vi "Release.vi"(8 "error in (no error)":errorcluster, 11 "[User] Cfg File in":refnum<class "[User] Cfg File.lvclass">) -> (0 "error out":errorcluster, 3 "[User] Cfg File out":refnum<class "[User] Cfg File.lvclass">)   [LabVIEW 2020, in "[User] Cfg File.lvclass"]
uses:
  [User] Cfg File.lvclass
  [User] Cfg File.lvclass/[User] Cfg File.ctl
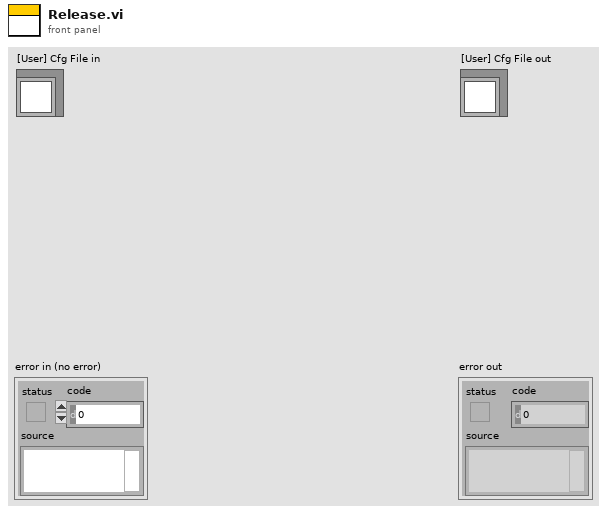
[diagram p1: front panel]
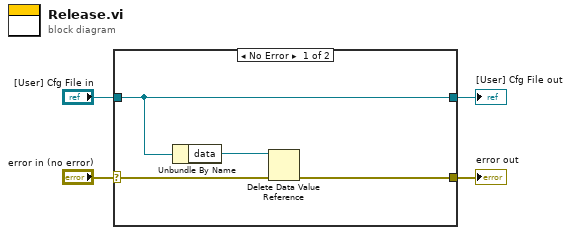
[diagram p0: block diagram]
diagram:
  n1 = case shown="No Error" "error in (no error)" {
    selector: "error in (no error)" -> [w7 w10]
    tunnel: [w5 w10] -> w3
    tunnel: [w8 w9] -> w1
    tunnel: "[User] Cfg File in" -> [w8 w9]
    frame No Error {
      n2 = Unbundle By Name(w8) -> ("data"=w6:refnum<data-value>)
      n3 = Delete Data Value Reference(data value reference=w6, error in=w7) -> (error out=w5:errorcluster)  [unwired: 1 out]
    }
    frame Error {
    }
  }
  "error out" <- w3
  "[User] Cfg File out" <- w1
